vi "FSK调制与解调.vi"() -> ()   [LabVIEW 2013]
uses:
  <vilib>/Analysis/3filter.llb/Butterworth Filter (DBL).vi
  <vilib>/express/express analysis/Spectral/Block/exnSpectralBlock spectral measurements peak poly.vi
  <vilib>/express/express analysis/Spectral/Block/exnSpectralBlock spectral measurements peak WFM.vi
  <vilib>/express/express analysis/Spectral/XNode/ExpressSpectralMeasurementsBlockNode.xnode
  <vilib>/Analysis/NI_AALBase.lvlib
panel:
  out "下路滤波后波形":dbl[](graph)
  out "上路滤波后波形":dbl[](graph)
  out "2FSK频谱图":cluster{"f0":dbl, "df":dbl, "magnitude":dbl[]}(graph)
  out "2FSK信号波形":dbl[](graph)
  out "载波2":dbl[](graph)
  out "载波1":dbl[](graph)
  out "输入序列波形":dbl[](graph)
  in  "噪声标准差":dbl
  out "一个码周期内的点数":dbl
  in  "码速率":dbl
  in  "载频2":dbl
  in  "载频1":dbl
  in  "载波相位":dbl
  in  "采样率":dbl
  in  "采样点数":i32
  out "输出序列":u32[](array[numeric])
  in  "输入序列":u32[](array[numeric]) format="%b"
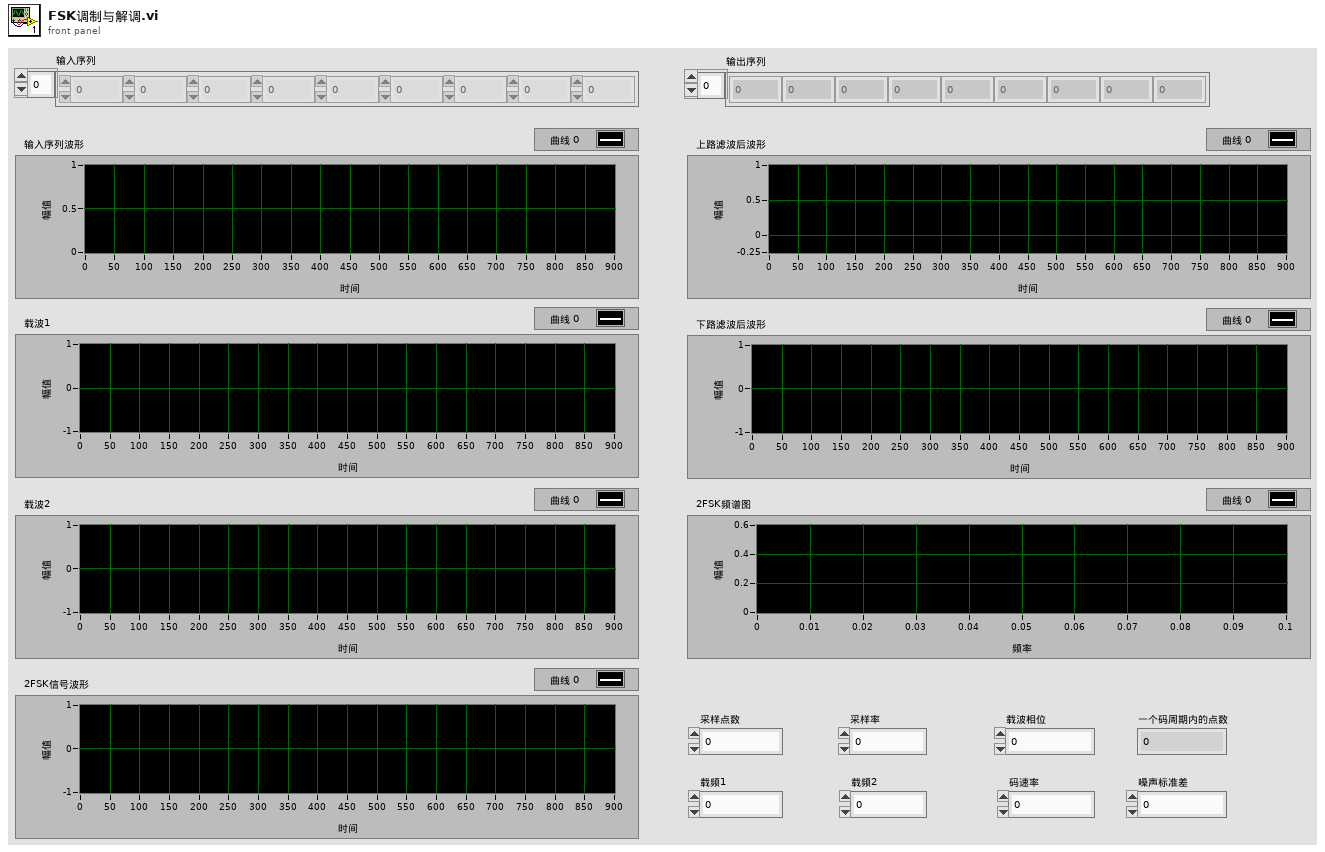
[diagram p1: front panel]
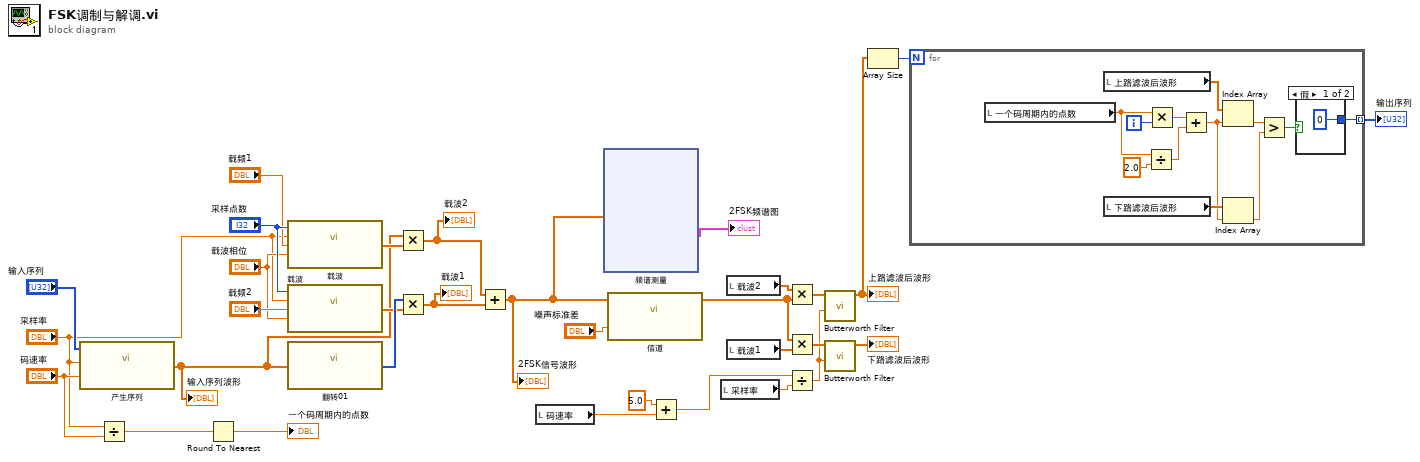
[diagram p0: block diagram]
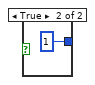
[diagram p2: hidden frame]
diagram:
  n1 = call "产生序列.vi"("码速率RB"="码速率", "采样率"="采样率", "输入序列"="输入序列") -> ("输入序列波形"=w20:dbl[])
  "输入序列波形" <- w20
  n2 = Divide(x="采样率", y="码速率") -> (x/y=w25:dbl)
  n3 = Round To Nearest(number=w25) -> (nearest integer value=→"一个码周期内的点数":dbl)
  n4 = call "载波.vi"("相位输入"="载波相位", "载频"="载频1", "采样率"="采样率", "采样点数"="采样点数") -> ("载波信号波形"=w21:dbl[])
  n5 = call "载波.vi"("相位输入"="载波相位", "载频"="载频2", "采样率"="采样率", "采样点数"="采样点数") -> ("载波信号波形"=w22:dbl[])
  n6 = call "翻转01.vi"("收到的信息序列"=w20) -> ("翻转后的波形"=w23:i32[])
  n7 = Multiply(x=w20, y=w21) -> (x*y=w4:dbl[])
  "载波2" <- w4
  n8 = Multiply(x=w23, y=w22) -> (x*y=w3:dbl[])
  "载波1" <- w3
  n9 = Add(x=w4, y=w3) -> (x+y=w1:dbl[])
  "2FSK信号波形" <- w1
  n10 = local read "码速率"() -> (w14:dbl)
  n11 = xnode "频谱测量"("信号"=w1) -> ("FFT - （峰值）"=→"2FSK频谱图":cluster{"f0":dbl, "df":dbl, "magnitude":dbl[]})  [unwired: 1 in, 2 out]
  n12 = call "信道.vi"("噪声标准差"="噪声标准差", "调制信号"=w1) -> ("信道输出信号"=w16:dbl[])  [unwired: 1 out]
  n13 = Add(x=5.0, y=w14) -> (x+y=w13:dbl)
  n14 = local read "采样率"() -> (w12:dbl)
  n15 = local read "载波2"() -> (w18:dbl[])
  n16 = local read "载波1"() -> (w17:dbl[])
  n17 = Multiply(x=w18, y=w16) -> (x*y=w11:dbl[])
  n18 = Multiply(x=w16, y=w17) -> (x*y=w10:dbl[])
  n19 = Divide(x=w13, y=w12) -> (x/y=w9:dbl)
  n20 = call-poly <vilib>:"Butterworth Filter.vi"("high cutoff freq: fh"=w9, "X"=w11) -> ("Filtered X"=w7:dbl[])  [unwired: 6 in, 1 out]
  "上路滤波后波形" <- w7
  n21 = call-poly <vilib>:"Butterworth Filter.vi"("high cutoff freq: fh"=w9, "X"=w10) -> ("Filtered X"=→"下路滤波后波形":dbl[])  [unwired: 6 in, 1 out]
  n22 = Array Size(array=w7) -> (size(s)=w6:i32)
  n23 = for {
    N: w6 -> [_]
    tunnel: [w35] -> w5 mode=indexing
    i -> [w44]
    n24 = local read "一个码周期内的点数"() -> (w41:dbl)
    n25 = local read "上路滤波后波形"() -> (w40:dbl[])
    n26 = local read "下路滤波后波形"() -> (w39:dbl[])
    n27 = Divide(x=w41, y=2.0) -> (x/y=w42:dbl)
    n28 = Multiply(x=w41, y=w44) -> (x*y=w34:dbl)
    n29 = Add(x=w34, y=w42) -> (x+y=w33:dbl)
    n30 = Index Array(array=w40, index=w33) -> (element=w38:dbl)
    n31 = Index Array(array=w39, index=w33) -> (element=w37:dbl)
    n32 = Greater?(x=w38, y=w37) -> (0:w36:bool)
    n33 = case shown="假" w36 {
      tunnel: [0 1] -> w35
      frame False {
      }
      frame True {
      }
    }
  }
  "输出序列" <- w5
